vi "Generate_WayPoints_WITHPAUSE.vi"(5 "Update Position Loop Wait Time (ms)":i16=-15536, 8 "Feedback Enum":u16=5, 11 "Input Cluster":T2={"Scan Rate (um/s)"=15.0, "X Start"=15.0, "X End"=15.0, "Y Start"=15.0, "Y End"=15.0, " Z Start"=15.0, "Number of Lines"=15, "V"=15.0, "Z End"=15.0, "Approach Rate (um/s)"=15.0, "Squish Approach Rate (um/s)"=15.0, "V 2"=15.0, "HoldTime / s"=15}) -> (0 "output cluster":T1)   [LabVIEW 2023]
uses:
  TypeDefs/WayPointCluster.ctl
  User_Vi/Settings.vi
panel:
  in  "WayPointCluster":T1
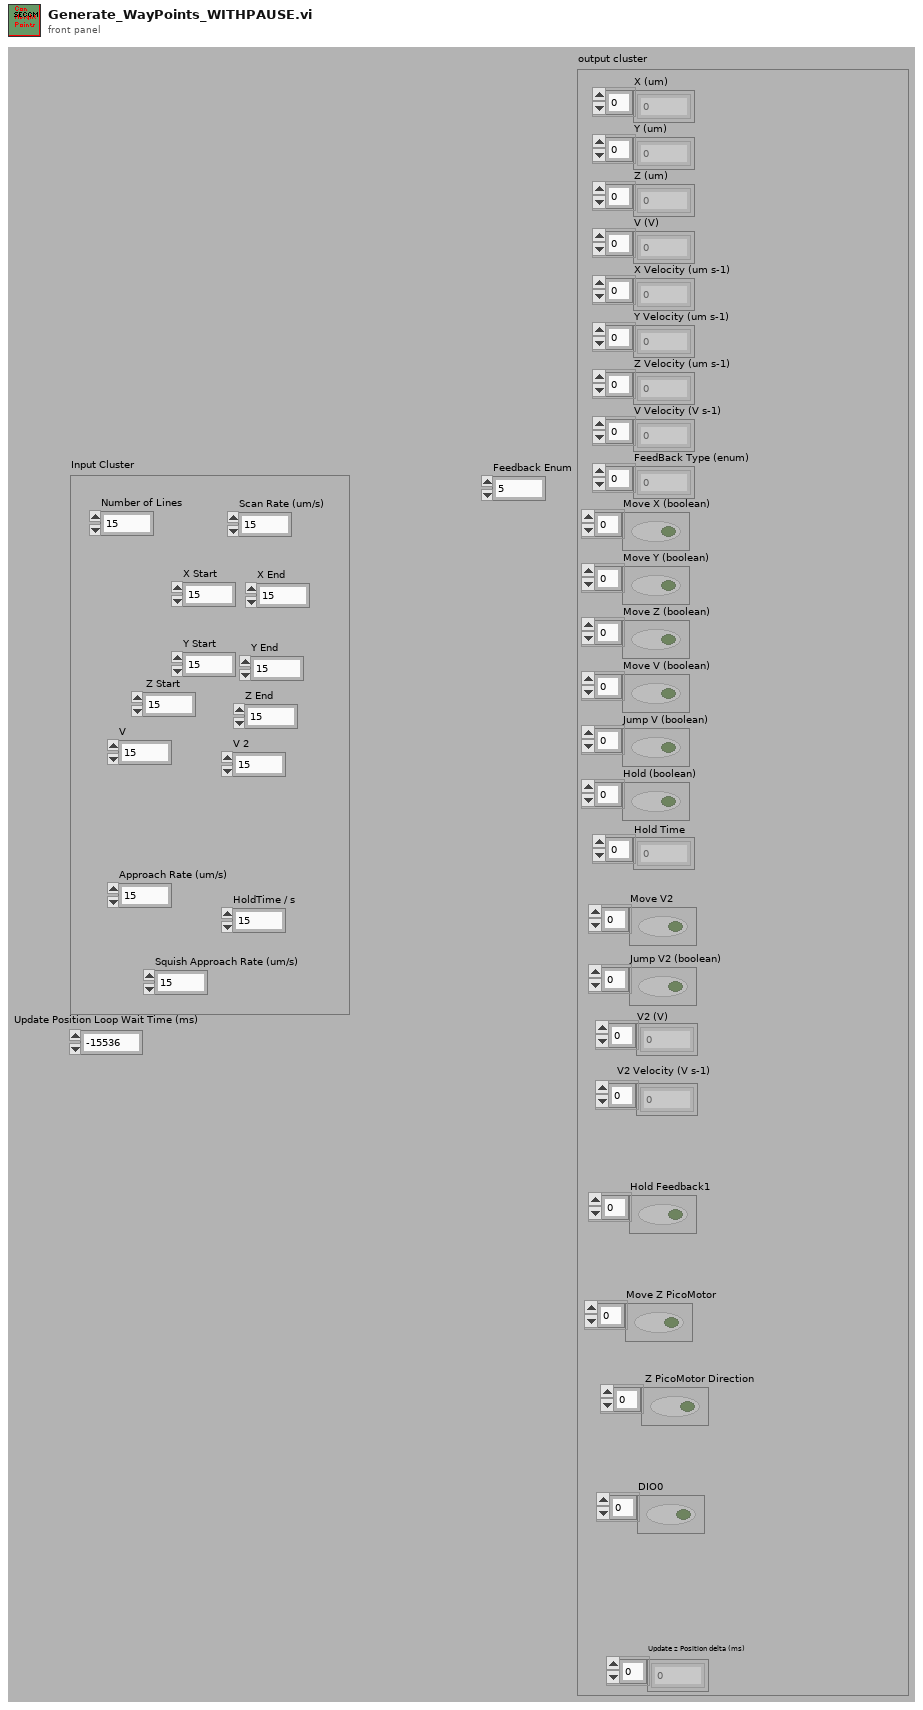
[diagram p1: front panel]
types:
  T1 = typedef "WayPointCluster.ctl" = cluster{"X (um)":dbl[], "Y (um)":dbl[], "Z (um)":dbl[], "V (V)":dbl[], "X Velocity (um s-1)":dbl[], "Y Velocity (um s-1)":dbl[], "Z Velocity (um s-1)":dbl[], "V Velocity (V s-1)":dbl[], "FeedBack Type (enum)":u16[], "Move X (boolean)":bool[], "Move Y (boolean)":bool[], "Move Z (boolean)":bool[], "Move V (boolean)":bool[], "Jump V (boolean)":bool[], "Hold (boolean)":bool[], "Hold Time":u32[], "V2 (V)":dbl[], "Move V2":bool[], "V2 Velocity (V s-1)":dbl[], "Jump V2 (boolean)":bool[], "Update z Position delta (ms)":i16[], "Hold Feedback1":bool[], "Move Z PicoMotor":bool[], " Z PicoMotor Direction":bool[], "DIO0":bool[]}
  T2 = cluster{"Scan Rate (um/s)":dbl, "X Start":dbl, "X End":dbl, "Y Start":dbl, "Y End":dbl, " Z Start":dbl, "Number of Lines":u32, "V":dbl, "Z End":dbl, "Approach Rate (um/s)":dbl, "Squish Approach Rate (um/s)":dbl, "V 2":dbl, "HoldTime / s":u32}
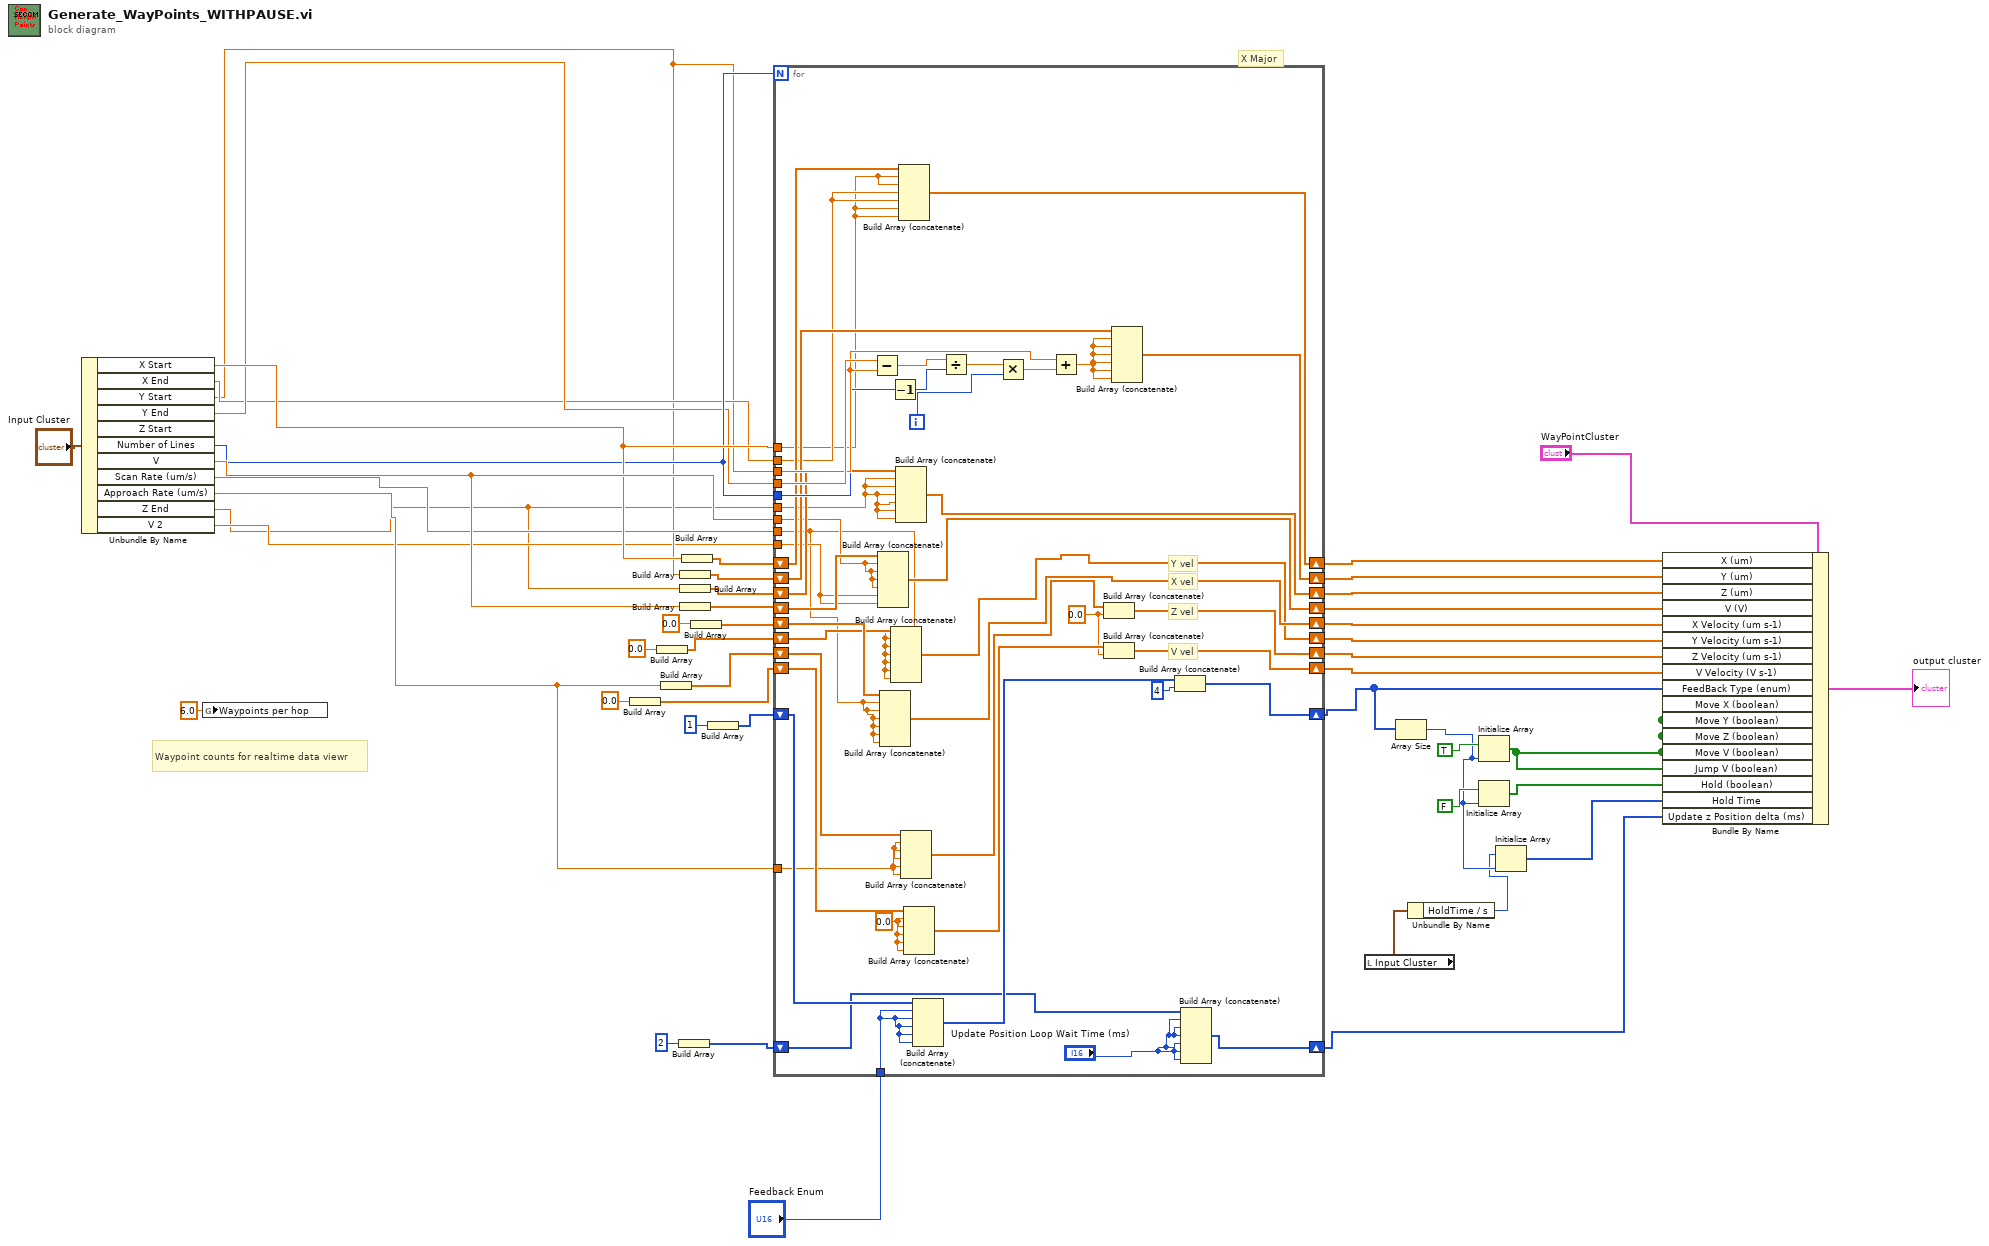
[diagram p0: block diagram]
diagram:
  # "Waypoint counts for realtime data viewr"
  # "X Major"
  n1 = Unbundle By Name("Input Cluster") -> ("X Start"=w46:dbl, "X End"=w33:dbl, "Y Start"=w32:dbl, "Y End"=w43:dbl, "Number of Lines"=w45:u32, "V"=w47:dbl, "Scan Rate (um/s)"=w44:dbl, "Approach Rate (um/s)"=w34:dbl, "Z End"=w2:dbl, "V 2"=w28:dbl)  [unwired: 1 out]
  n2 = global write "Settings.vi" "Waypoints per hop"(6.0 ("Waypoints per hop")) -> ()
  n3 = Build Array(0.0 ("element")) -> (w14:dbl[])
  n4 = Build Array(0.0 ("element")) -> (w11:dbl[])
  n5 = Build Array(w34) -> (w13:dbl[])
  n6 = Build Array(i16 2 ("element")) -> (w3:i16[])
  n7 = Build Array(w32) -> (w6:dbl[])
  n8 = Build Array(w2) -> (w7:dbl[])
  n9 = Build Array(w47) -> (w9:dbl[])
  n10 = Build Array(w46) -> (w5:dbl[])
  n11 = Build Array(0.0 ("element")) -> (w10:dbl[])
  n12 = Build Array(u16 1 ("element")) -> (w16:u16[])
  n13 = for {
    N: w45 -> [_]
    tunnel: w46 -> [w65]
    tunnel: w33 -> [w66]
    tunnel: w2 -> [w62]
    tunnel: w47 -> [w61]
    tunnel: w32 -> [w91]
    tunnel: w43 -> [w92]
    tunnel: w45 -> [w87]
    tunnel: w44 -> [w54]
    shift-right: [w56] -> w42
    shift-left: w10 -> [w86]
    shift-right: [w77] -> w37
    shift-left: w6 -> [w85]
    shift-right: [w75] -> w35
    shift-left: w9 -> [w67]
    shift-right: [w78] -> w41
    shift-left: w5 -> [w84]
    shift-right: [w76] -> w36
    shift-left: w7 -> [w83]
    shift-right: [w55] -> w40
    shift-left: w11 -> [w82]
    shift-right: [w71] -> w38
    shift-left: w13 -> [w81]
    shift-right: [w72] -> w39
    shift-left: w14 -> [w80]
    shift-right: [w68] -> w30
    shift-left: w16 -> [w70]
    tunnel: w28 -> [w60]
    tunnel: w34 -> [w53]
    tunnel: "Feedback Enum" -> [w52]
    shift-right: [w50] -> w18
    shift-left: w3 -> [w51]
    i -> [w63]
    w58 = 0.0 ("element")
    w59 = 0.0 ("element")
    # "Y vel"
    # "X vel"
    # "Z vel"
    # "V vel"
    n14 = Subtract(x=w92, y=w91) -> (x-y=w90:dbl)
    n15 = Build Array (concatenate)(w67, w61, w61, w61, w61, w60, w60) -> (w75:dbl[])
    n16 = Build Array (concatenate)(w86, w54, w54, w54, w54, w54, w54) -> (w56:dbl[])
    n17 = Decrement(x=w87) -> (x-1=w79:u32)
    n18 = Build Array (concatenate)(w82, w54, w54, w54, w54, w54, w54) -> (w55:dbl[])
    n19 = Build Array (concatenate)(w83, w62, w62, w62, w62, w62, w62) -> (w76:dbl[])
    n20 = Build Array (concatenate)(w84, w65, w65, w66, w66, w65, w65) -> (w78:dbl[])
    n21 = Build Array (concatenate)(w81, w53, w53, w53, w53, w53) -> (w74:dbl[])
    n22 = Build Array (concatenate)(w80, w59, w59, w59, w59, w59) -> (w73:dbl[])
    n23 = Build Array (concatenate)(w70, w52, w52, w52, w52, w52) -> (w69:u16[])
    n24 = Divide(x=w90, y=w79) -> (x/y=w88:dbl)
    n25 = Multiply(x=w88, y=w63) -> (x*y=w89:dbl)
    n26 = Add(x=w91, y=w89) -> (x+y=w64:dbl)
    n27 = Build Array (concatenate)(w74, w58) -> (w71:dbl[])
    n28 = Build Array (concatenate)(w73, w58) -> (w72:dbl[])
    n29 = Build Array (concatenate)(w85, w64, w64, w64, w64, w64, w64) -> (w77:dbl[])
    n30 = Build Array (concatenate)(w69, u16 4 ("element")) -> (w68:u16[])
    n31 = Build Array (concatenate)(w51, "Update Position Loop Wait Time (ms)", "Update Position Loop Wait Time (ms)", "Update Position Loop Wait Time (ms)", "Update Position Loop Wait Time (ms)", "Update Position Loop Wait Time (ms)", "Update Position Loop Wait Time (ms)") -> (w50:i16[])
  }
  n32 = local read "Input Cluster"() -> (w24:T2)
  n33 = Array Size(array=w30) -> (size(s)=w25:i32)
  n34 = Unbundle By Name(w24) -> ("HoldTime / s"=w23:u32)
  n35 = Initialize Array(TRUE, w25) -> (w29:bool[])
  n36 = Initialize Array(FALSE, w25) -> (w26:bool[])
  n37 = Initialize Array(w23, w25) -> (w22:u32[])
  n38 = Bundle By Name(cluster="WayPointCluster", "X (um)"=w41, "Y (um)"=w37, "Z (um)"=w36, "V (V)"=w35, "X Velocity (um s-1)"=w42, "Y Velocity (um s-1)"=w40, "Z Velocity (um s-1)"=w38, "V Velocity (V s-1)"=w39, "FeedBack Type (enum)"=w30, "Move X (boolean)"=w29, "Move Y (boolean)"=w29, "Move Z (boolean)"=w29, "Move V (boolean)"=w29, "Jump V (boolean)"=w29, "Hold (boolean)"=w26, "Hold Time"=w22, "Update z Position delta (ms)"=w18) -> (→"output cluster":T1)
